vi "writeTSVariable(string).vi"(0 "Engine Reference":refnum<k7>, 5 "Sequence File Ref":refnum<k7>, 7 "Variable Type":i32(ring)=1 items=["PropValType_Container", "PropValType_String", "PropValType_Boolean", "PropValType_Number", "PropValType_NamedType", "PropValType_Reference", "PropValType_Array"], 9 "Variable Name":string="Locals.Logs", 11 "error in":errorcluster, 12 "newValue":string) -> (4 "Engine Reference(out)":refnum<k7>, 6 "Sequence File Ref(out)":refnum<k7>, 15 "error out":errorcluster)   [LabVIEW 2009]
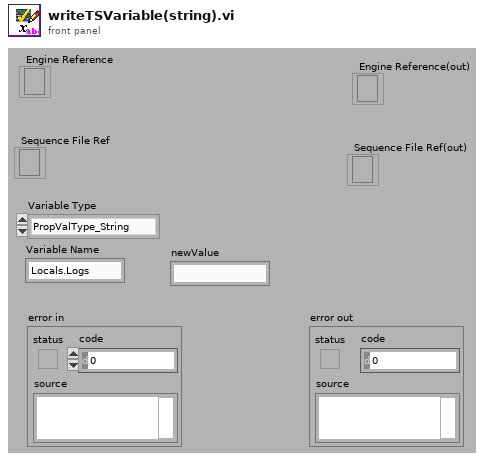
[diagram p1: front panel]
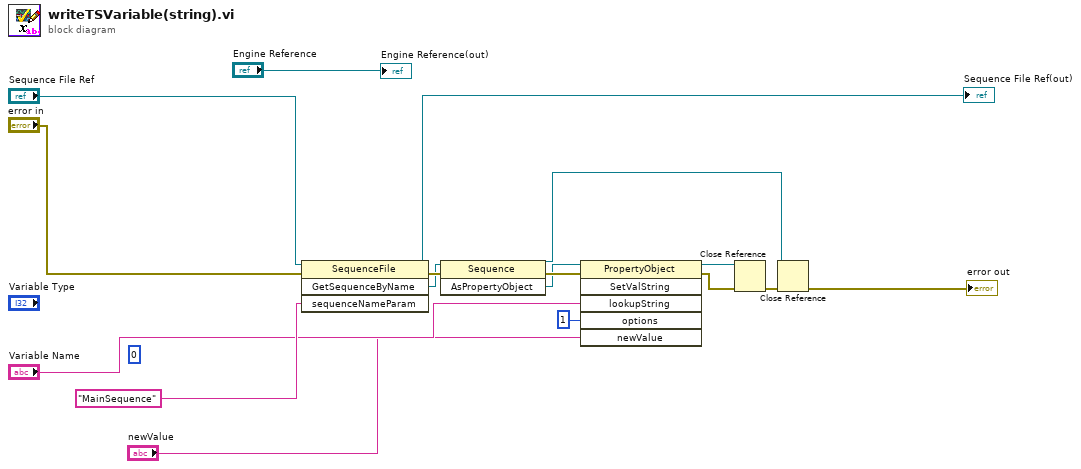
[diagram p0: block diagram]
diagram:
  (unwired) 0 ("options")
  n1 = invoke class="SequenceFile" method="GetSequenceByName"(reference="Sequence File Ref", error in="error in", "sequenceNameParam"="MainSequence") -> (reference out=→"Sequence File Ref(out)":refnum<k7>, error out=w13:errorcluster, "GetSequenceByName"=w11:refnum<k7>)  [unwired: 1 in, 1 out]
  n2 = invoke class="Sequence" method="AsPropertyObject"(reference=w11, error in=w13) -> (reference out=w15:refnum<k7>, error out=w9:errorcluster, "AsPropertyObject"=w8:refnum<k7>)  [unwired: 1 in]
  n3 = invoke class="PropertyObject" method="SetValString"(reference=w8, error in=w9, "lookupString"="Variable Name", "options"=1, "newValue"="newValue") -> (reference out=w3:refnum<k7>, error out=w2:errorcluster)  [unwired: 1 in, 4 out]
  n4 = Close Reference(reference=w3, error in (no error)=w2) -> (error out=w14:errorcluster)
  n5 = Close Reference(reference=w15, error in (no error)=w14) -> (error out=→"error out":errorcluster)
  "Engine Reference(out)" <- "Engine Reference"
